vi "Input Entry Resize.vi"(8 "NewBnds":T2, 10 "Refnums":T1, 11 "Control Refnum in":refnum<vi>) -> (3 "Control Refnum out":refnum<vi>)   [LabVIEW 2015, in "CallVIStep.lvclass"]
uses:
  CallVIStep.lvclass
  <vilib>/Utility/miscctls.llb/LVRectTypeDef.ctl
  VI Input Type Typedef.ctl
  <vilib>/Utility/miscctls.llb/LVPositionTypeDef.ctl
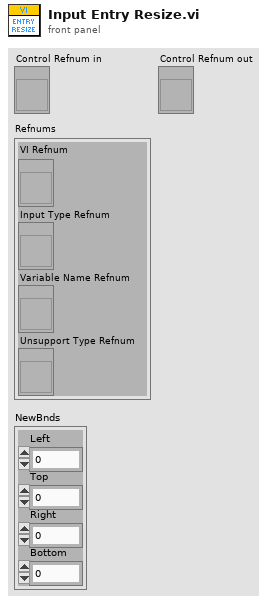
[diagram p1: front panel]
types:
  T1 = cluster{"VI Refnum":refnum<vi>, "Input Type Refnum":refnum<vi>, "Variable Name Refnum":refnum<vi>, "Unsupport Type Refnum":refnum<vi>}
  T2 = typedef "LVRectTypeDef.ctl" = cluster{"Left":i16, "Top":i16, "Right":i16, "Bottom":i16}
  T3 = typedef "LVPositionTypeDef.ctl" = cluster{"Left":i32, "Top":i32}
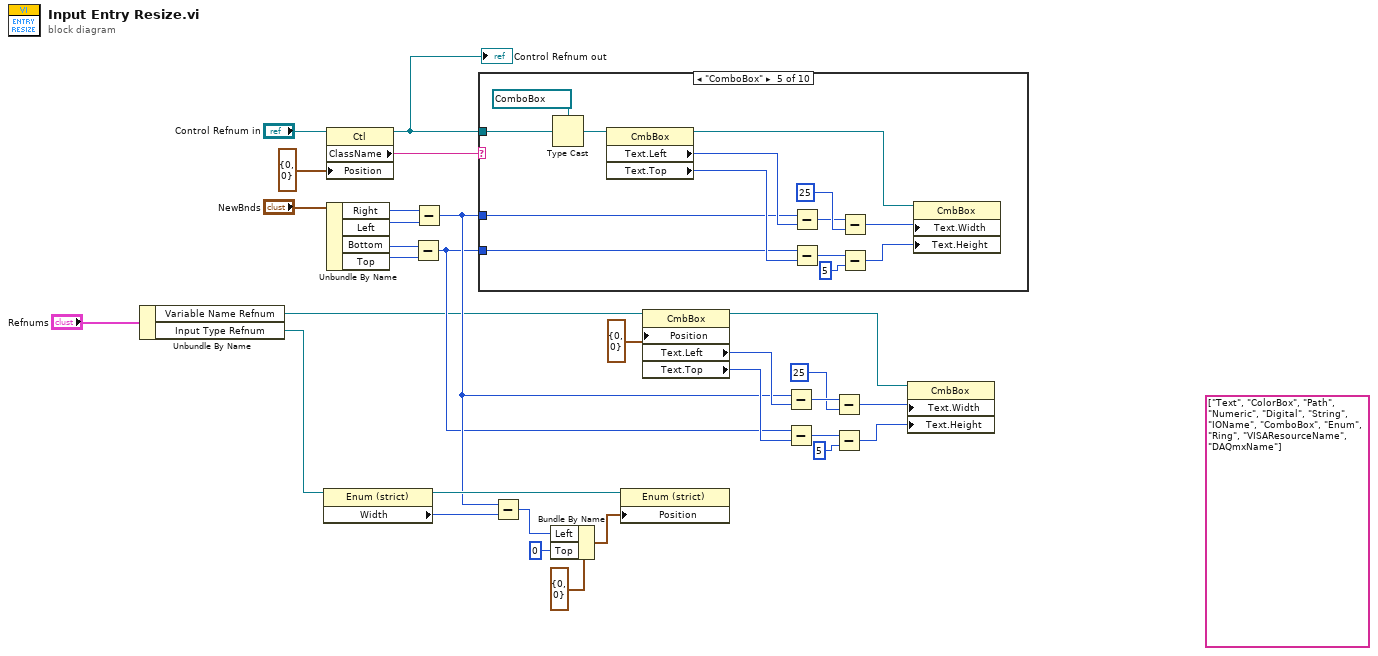
[diagram p0: block diagram]
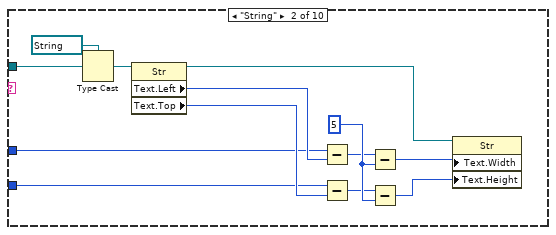
[diagram p3: hidden frame]
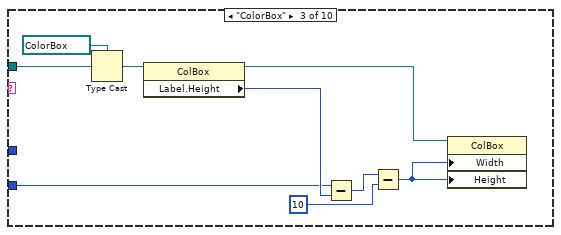
[diagram p4: hidden frame]
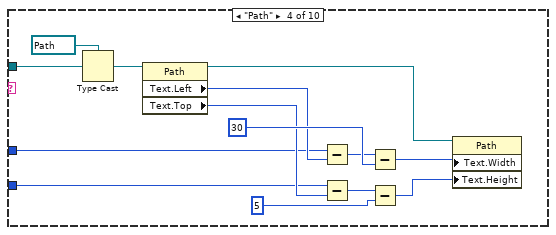
[diagram p5: hidden frame]
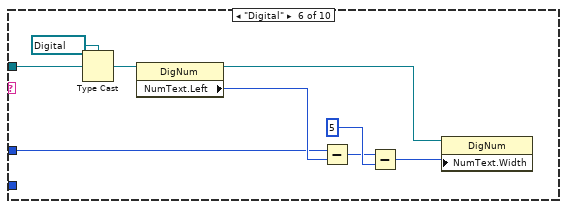
[diagram p6: hidden frame]
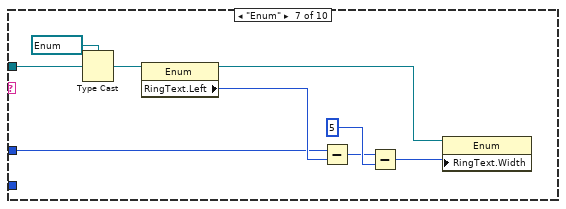
[diagram p7: hidden frame]
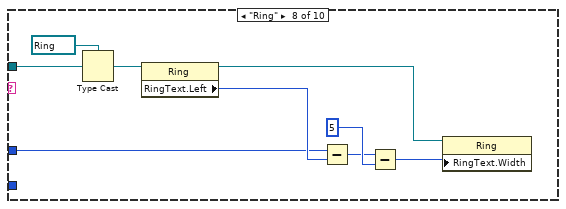
[diagram p8: hidden frame]
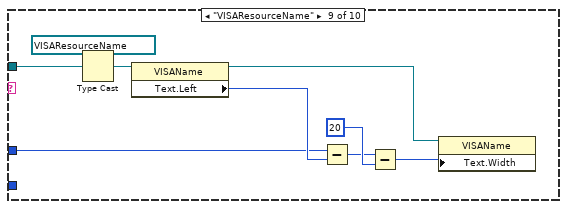
[diagram p9: hidden frame]
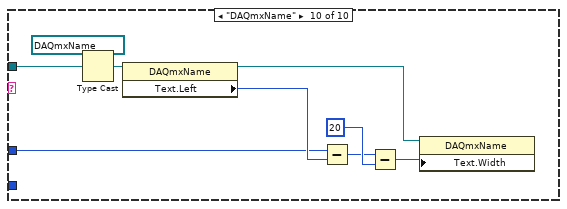
[diagram p10: hidden frame]
diagram:
  (unwired) string[] ["Text", "ColorBox", "Path", "Numeric", "Digital", "String", "IOName", "ComboBox", "Enum", "Ring", "VISAResourceName", "DAQmxName"] ("Strings []")
  n1 = Unbundle By Name("Refnums") -> ("Variable Name Refnum"=w2:refnum<vi>, "Input Type Refnum"=w1:refnum<vi>)
  n2 = property class="Enum (strict)"(reference=w1) -> (reference out=w23:refnum<vi>, "Width"=w22:u32)  [unwired: 1 in, 1 out]
  n3 = property class="Ctl"(reference="Control Refnum in", "Position"=T3 {"Left"=0, "Top"=0}) -> (reference out=w17:refnum<vi>, "ClassName"=w19:string)  [unwired: 1 in, 1 out]
  "Control Refnum out" <- w17
  n4 = Unbundle By Name("NewBnds") -> ("Right"=w29:i16, "Left"=w28:i16, "Bottom"=w27:i16, "Top"=w26:i16)
  n5 = Subtract(x=w27, y=w26) -> (x-y=w5:i16)
  n6 = Subtract(x=w29, y=w28) -> (x-y=w6:i16)
  n7 = case shown="\"ComboBox\"" w19 {
    tunnel: w5 -> [_ w37 w47 w60 w74 _ _ _ _ _]
    tunnel: w17 -> [_ w33 w51 w56 w70 w83 w92 w101 w110 w119]
    tunnel: w6 -> [_ w34 _ w57 w71 w84 w93 w102 w111 w120]
    frame Default {
    }
    frame "String" {
      w42 = 5
      n8 = Type Cast(type=refnum<vi> refnum ("String in"), x=w33) -> (*(type *) &x=w31:refnum<vi>)
      n9 = property class="Str"(reference=w31) -> (reference out=w35:refnum<vi>, "Text.Left"=w36:i32, "Text.Top"=w38:i32)  [unwired: 1 in, 1 out]
      n10 = Subtract(x=w34, y=w36) -> (x-y=w39:i32)
      n11 = Subtract(x=w37, y=w38) -> (x-y=w41:i32)
      n12 = Subtract(x=w39, y=w42) -> (x-y=w40:i32)
      n13 = Subtract(x=w41, y=w42) -> (x-y=w43:i32)
      n14 = property class="Str"(reference=w35, "Text.Width"=w40, "Text.Height"=w43) -> ()  [unwired: 1 in, 2 out]
    }
    frame "ColorBox" {
      n15 = Type Cast(type=refnum<vi> refnum ("String in"), x=w51) -> (*(type *) &x=w49:refnum<vi>)
      n16 = property class="ColBox"(reference=w49) -> (reference out=w52:refnum<vi>, "Label.Height"=w48:u32)  [unwired: 1 in, 1 out]
      n17 = Subtract(x=w47, y=w48) -> (x-y=w46:u32)
      n18 = Subtract(x=w46, y=10) -> (x-y=w44:u32)
      n19 = property class="ColBox"(reference=w52, "Width"=w44, "Height"=w44) -> ()  [unwired: 1 in, 2 out]
    }
    frame "Path" {
      n20 = Type Cast(type=refnum<vi> refnum ("String in"), x=w56) -> (*(type *) &x=w54:refnum<vi>)
      n21 = property class="Path"(reference=w54) -> (reference out=w58:refnum<vi>, "Text.Left"=w59:i32, "Text.Top"=w61:i32)  [unwired: 1 in, 1 out]
      n22 = Subtract(x=w57, y=w59) -> (x-y=w62:i32)
      n23 = Subtract(x=w60, y=w61) -> (x-y=w64:i32)
      n24 = Subtract(x=w62, y=30) -> (x-y=w63:i32)
      n25 = Subtract(x=w64, y=5) -> (x-y=w66:i32)
      n26 = property class="Path"(reference=w58, "Text.Width"=w63, "Text.Height"=w66) -> ()  [unwired: 1 in, 2 out]
    }
    frame "ComboBox" {
      n27 = Type Cast(type=refnum<vi> refnum ("String in"), x=w70) -> (*(type *) &x=w68:refnum<vi>)
      n28 = property class="CmbBox"(reference=w68) -> (reference out=w72:refnum<vi>, "Text.Left"=w73:i32, "Text.Top"=w75:i32)  [unwired: 1 in, 1 out]
      n29 = Subtract(x=w71, y=w73) -> (x-y=w76:i32)
      n30 = Subtract(x=w74, y=w75) -> (x-y=w78:i32)
      n31 = Subtract(x=w76, y=25) -> (x-y=w77:i32)
      n32 = Subtract(x=w78, y=5) -> (x-y=w80:i32)
      n33 = property class="CmbBox"(reference=w72, "Text.Width"=w77, "Text.Height"=w80) -> ()  [unwired: 1 in, 2 out]
    }
    frame "Digital" {
      n34 = Type Cast(type=refnum<vi> refnum ("String in"), x=w83) -> (*(type *) &x=w81:refnum<vi>)
      n35 = property class="DigNum"(reference=w81) -> (reference out=w85:refnum<vi>, "NumText.Left"=w86:i32)  [unwired: 1 in, 1 out]
      n36 = Subtract(x=w84, y=w86) -> (x-y=w87:i32)
      n37 = Subtract(x=w87, y=5) -> (x-y=w88:i32)
      n38 = property class="DigNum"(reference=w85, "NumText.Width"=w88) -> ()  [unwired: 1 in, 2 out]
    }
    frame "Enum" {
      n39 = Type Cast(type=refnum<vi> refnum ("String in"), x=w92) -> (*(type *) &x=w90:refnum<vi>)
      n40 = property class="Enum"(reference=w90) -> (reference out=w94:refnum<vi>, "RingText.Left"=w95:i32)  [unwired: 1 in, 1 out]
      n41 = Subtract(x=w93, y=w95) -> (x-y=w96:i32)
      n42 = Subtract(x=w96, y=5) -> (x-y=w97:i32)
      n43 = property class="Enum"(reference=w94, "RingText.Width"=w97) -> ()  [unwired: 1 in, 2 out]
    }
    frame "Ring" {
      n44 = Type Cast(type=refnum<vi> refnum ("String in"), x=w101) -> (*(type *) &x=w99:refnum<vi>)
      n45 = property class="Ring"(reference=w99) -> (reference out=w103:refnum<vi>, "RingText.Left"=w104:i32)  [unwired: 1 in, 1 out]
      n46 = Subtract(x=w102, y=w104) -> (x-y=w105:i32)
      n47 = Subtract(x=w105, y=5) -> (x-y=w106:i32)
      n48 = property class="Ring"(reference=w103, "RingText.Width"=w106) -> ()  [unwired: 1 in, 2 out]
    }
    frame "VISAResourceName" {
      n49 = Type Cast(type=refnum<vi> refnum ("String in"), x=w110) -> (*(type *) &x=w108:refnum<vi>)
      n50 = property class="VISAName"(reference=w108) -> (reference out=w112:refnum<vi>, "Text.Left"=w113:i32)  [unwired: 1 in, 1 out]
      n51 = Subtract(x=w111, y=w113) -> (x-y=w114:i32)
      n52 = Subtract(x=w114, y=20) -> (x-y=w115:i32)
      n53 = property class="VISAName"(reference=w112, "Text.Width"=w115) -> ()  [unwired: 1 in, 2 out]
    }
    frame "DAQmxName" {
      n54 = Type Cast(type=refnum<vi> refnum ("String in"), x=w119) -> (*(type *) &x=w117:refnum<vi>)
      n55 = property class="DAQmxName"(reference=w117) -> (reference out=w121:refnum<vi>, "Text.Left"=w122:i32)  [unwired: 1 in, 1 out]
      n56 = Subtract(x=w120, y=w122) -> (x-y=w123:i32)
      n57 = Subtract(x=w123, y=20) -> (x-y=w124:i32)
      n58 = property class="DAQmxName"(reference=w121, "Text.Width"=w124) -> ()  [unwired: 1 in, 2 out]
    }
  }
  n59 = Subtract(x=w6, y=w22) -> (x-y=w16:u32)
  n60 = Bundle By Name(cluster=T3 {"Left"=0, "Top"=0} ("Position"), "Left"=w16, "Top"=0) -> (w24:T3)
  n61 = property class="Enum (strict)"(reference=w23, "Position"=w24) -> ()  [unwired: 1 in, 2 out]
  n62 = property class="CmbBox"(reference=w2, "Position"=T3 {"Left"=0, "Top"=0} ("Text.Position")) -> (reference out=w14:refnum<vi>, "Text.Left"=w13:i32, "Text.Top"=w12:i32)  [unwired: 1 in, 1 out]
  n63 = Subtract(x=w6, y=w13) -> (x-y=w11:i32)
  n64 = Subtract(x=w5, y=w12) -> (x-y=w9:i32)
  n65 = Subtract(x=w11, y=25) -> (x-y=w10:i32)
  n66 = Subtract(x=w9, y=5) -> (x-y=w7:i32)
  n67 = property class="CmbBox"(reference=w14, "Text.Width"=w10, "Text.Height"=w7) -> ()  [unwired: 1 in, 2 out]
